vi "SIM Ros Find k3.vi"(2 "Ros data":T1, 3 "step size":dbl, 4 "F2":dbl[](array[numeric])) -> (0 "Error?":bool, 1 "k":dbl[](array[numeric]))   [LabVIEW 2020]
uses:
  SIM Rosenbrock data.ctl
  SIM Factored Matrix.ctl
  SIM Ros stages.ctl
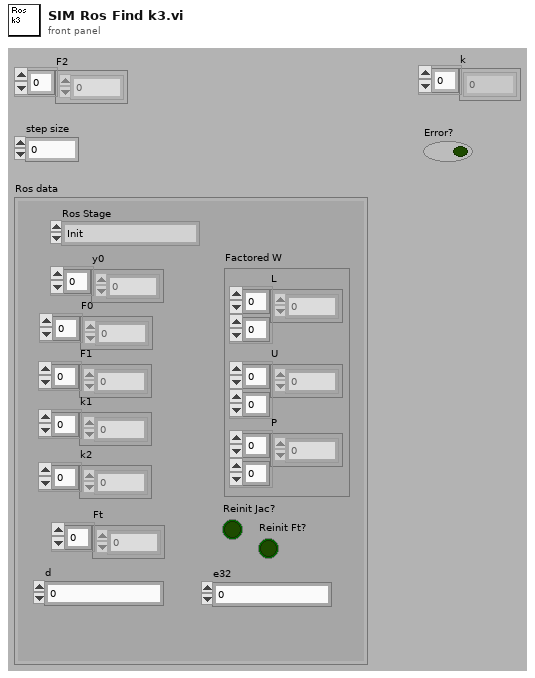
[diagram p1: front panel]
types:
  T1 = typedef "SIM Rosenbrock data.ctl" = cluster{"y0":dbl[], "F0":dbl[], "F1":dbl[], "k1":dbl[], "k2":dbl[], "Factored W":T2, "Ros Stage":T3, "Ft":dbl[], "Reinit Jac?":bool, "Reinit Ft?":bool, "d":dbl, "e32":dbl}
  T2 = typedef "SIM Factored Matrix.ctl" = cluster{"L":dbl[][], "U":dbl[][], "P":i32[][]}
  T3 = typedef "SIM Ros stages.ctl" = enum16{"Init", "Compute Jacobian", "Compute Ft", "Compute k1", "Compute k2", "Eval Error", "Choose StepSize", "Reset Integrator"}
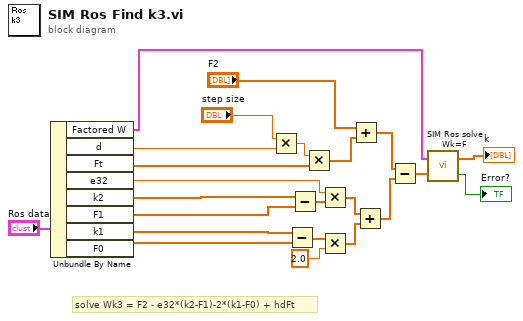
[diagram p0: block diagram]
diagram:
  # "solve Wk3 = F2 - e32*(k2-F1)-2*(k1-F0) + hdFt"
  n1 = Unbundle By Name("Ros data") -> ("Factored W"=w1:T2, "d"=w13:dbl, "Ft"=w11:dbl[], "e32"=w8:dbl, "k2"=w3:dbl[], "F1"=w4:dbl[], "k1"=w5:dbl[], "F0"=w6:dbl[])
  n2 = Multiply(x="step size", y=w13) -> (x*y=w14:dbl)
  n3 = Subtract(x=w5, y=w6) -> (x-y=w9:dbl[])
  n4 = Subtract(x=w3, y=w4) -> (x-y=w7:dbl[])
  n5 = Multiply(x=w14, y=w11) -> (x*y=w18:dbl[])
  n6 = Multiply(x=w8, y=w7) -> (x*y=w15:dbl[])
  n7 = Multiply(x=w9, y=2.0) -> (x*y=w16:dbl[])
  n8 = Add(x="F2", y=w18) -> (x+y=w19:dbl[])
  n9 = Add(x=w15, y=w16) -> (x+y=w20:dbl[])
  n10 = Subtract(x=w19, y=w20) -> (x-y=w21:dbl[])
  n11 = call "SIM Ros solve Wk=F.vi"("F"=w21, "Factored W"=w1) -> ("Error?"=→"Error?":bool, "k"=→"k":dbl[])
